vi "aod_calc_scale_digital.vi"(8 "FPGA parameters in":T1 {"AOD center frequ. (Hz)_y" format="%.14g"; "AOD half bandwidth_y" format="%.14g"; "AOD Bandwidth_y (Hz)" format="%_6f"; "AOD center frequ. (Hz)_x" format="%.14g"; "cos Phi" format="%.35g"; "sin Phi" format="%.35g"; "AOD_Scale_Factor (1/Zoom)" format="%.35g"; "AOD half bandwidth_x" format="%.14g"; "AOD Bandwidth_x (Hz)" format="%_6f"}, 9 "channel selector in":enum16{"x-channel", "y-channel"}(ring), 10 "acquire?":bool, 11 "input":fxp<+/-,36,32> format="%.14g") -> (0 "FPGA parameters out":T1 {"AOD center frequ. (Hz)_y" format="%.14g"; "AOD half bandwidth_y" format="%.14g"; "AOD Bandwidth_y (Hz)" format="%_6f"; "AOD center frequ. (Hz)_x" format="%.14g"; "cos Phi" format="%.35g"; "sin Phi" format="%.35g"; "AOD_Scale_Factor (1/Zoom)" format="%.35g"; "AOD half bandwidth_x" format="%.14g"; "AOD Bandwidth_x (Hz)" format="%_6f"}, 3 "output":fxp<+,36,32> format="%.14g")   [LabVIEW 2010]
uses:
  FPGA_parameters_cluster.ctl
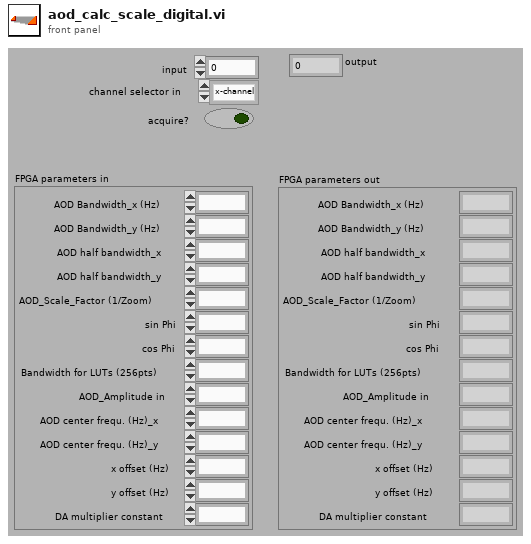
[diagram p1: front panel]
types:
  T1 = typedef "FPGA_parameters_cluster.ctl" = cluster{"AOD Bandwidth_x (Hz)":fxp<+,36,32>, "AOD Bandwidth_y (Hz)":fxp<+,36,32>, "AOD half bandwidth_x":fxp<+,36,32>, "AOD half bandwidth_y":fxp<+,36,32>, "AOD_Scale_Factor (1/Zoom)":fxp<+,36,2>, "sin Phi":fxp<+/-,36,2>, "cos Phi":fxp<+/-,36,2>, "Bandwidth for LUTs (256pts)":fxp<+,36,0>, "AOD_Amplitude in":u16, "AOD center frequ. (Hz)_x":fxp<+,36,32>, "AOD center frequ. (Hz)_y":fxp<+,36,32>, "x offset (Hz)":fxp<+/-,36,32>, "y offset (Hz)":fxp<+/-,36,32>, "DA multiplier constant":fxp<+,64,4>}
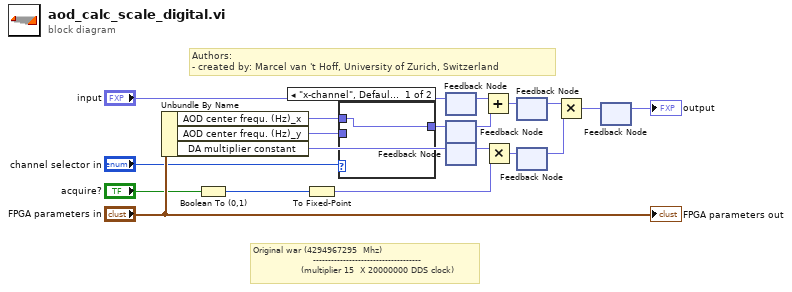
[diagram p0: block diagram]
diagram:
  # "Authors: \n- created by: Marcel van 't Hoff, University of Zurich, Switzerland"
  # "Original war (4294967295  Mhz)\n                    ------------------------------------\n                (multiplier 15  X 20000000 DDS clock)"
  n1 = Unbundle By Name("FPGA parameters in") -> ("AOD center frequ. (Hz)_x"=w11:fxp<+,36,32>, "AOD center frequ. (Hz)_y"=w9:fxp<+,36,32>, "DA multiplier constant"=w2:fxp<+,64,4>)
  n2 = Boolean To (0,1)(Boolean="acquire?") -> (0, 1=w3:i16)
  n3 = To Fixed-Point(number=w3) -> (fixed-point=w4:fxp<+,1,1>)  [unwired: 1 in]
  n4 = case shown="\"x-channel\", Default" "channel selector in" {
    tunnel: w11 -> [w20 _]
    tunnel: [w20 w21] -> w10
    tunnel: w9 -> [_ w21]
    frame "x-channel", Default {
    }
    frame "y-channel" {
    }
  }
  n5 = feedback-in #1("input") -> ()
  n6 = feedback #1() -> (w18:fxp<+/-,36,32>)  [unwired: 1 out]
  n7 = feedback-in #2(w10) -> ()
  n8 = feedback #2() -> (w15:fxp<+,36,32>)  [unwired: 1 out]
  n9 = feedback-in #3(w2) -> ()
  n10 = feedback #3() -> (w7:fxp<+,64,4>)  [unwired: 1 out]
  n11 = Add(x=w18, y=w15) -> (x+y=w19:fxp<+,36,32>)
  n12 = Multiply(x=w7, y=w4) -> (x*y=w5:fxp<+,64,4>)
  n13 = feedback-in #4(w19) -> ()
  n14 = feedback #4() -> (w17:fxp<+,36,32>)  [unwired: 1 out]
  n15 = feedback-in #5(w5) -> ()
  n16 = feedback #5() -> (w14:fxp<+,64,4>)  [unwired: 1 out]
  n17 = Multiply(x=w17, y=w14) -> (x*y=w1:fxp<+,36,32>)
  n18 = feedback-in #6(w1) -> ()
  n19 = feedback #6() -> (→"output":fxp<+,36,32>)  [unwired: 1 out]
  "FPGA parameters out" <- "FPGA parameters in"
